vi "Teleop.vi"(10 "Match Info":T1={"Autonomous Elapsed Seconds"=0.0, "TeleOp Elapsed Seconds"=0.0, "Disabled Elapsed Seconds"=0.0, "Visited Autonomous"=FALSE, "Visited TeleOp"=FALSE, "Visited Disabled"=FALSE, "Autonomous Settings"={"Autonomous Style"=enum."Independent", "VI Refnum"=refnum}}, 11 "Call Context":T2) -> ()   [LabVIEW 2013]
doc: "This VI is called for each TeleOp packet received from the DS where the robot is not disabled. It is often used to read from the joysticks and update I/O or to update setpoints for timed control loops. It should complete and return within 20 milliseconds or it may miss DS packets."
uses:
  Robot Global Data.vi
  <vilib>/Rock Robotics/WPI/Joystick/WPI_JoystickDeviceEnum.ctl
  <vilib>/Rock Robotics/WPI/Joystick/WPI_JoystickDevRef.ctl
  <vilib>/Rock Robotics/SystemInterfaces/DIO/FPGA_DIOChannel.ctl
  <vilib>/Rock Robotics/SystemInterfaces/Typedef/FPGA_TypedefDigitalModule.ctl
  <vilib>/Rock Robotics/WPI/DigitalInput/WPI_DigitalInputDevRef.ctl
  <vilib>/Rock Robotics/WPI/RobotDrive/WPI_RobotDriveMecanumDrive_Cartesian.vi
  <vilib>/Rock Robotics/SystemInterfaces/DIO/FPGA_DIORelayChannel.ctl
  <vilib>/Rock Robotics/WPI/Relay/WPI_RelayDirection.ctl
  <vilib>/Rock Robotics/WPI/Relay/WPI_RelayDevRef.ctl
  <vilib>/Rock Robotics/WPI/Relay/WPI_RelayValue.ctl
  <vilib>/Rock Robotics/WPI/DriverStation/WPI_DriverStationMatch Info.ctl
  <vilib>/Rock Robotics/WPI/DriverStation/WPI_DriverStationDerivedRobotMode.ctl
panel:
  out "Right Belt":dbl
  out "Left Belt":dbl
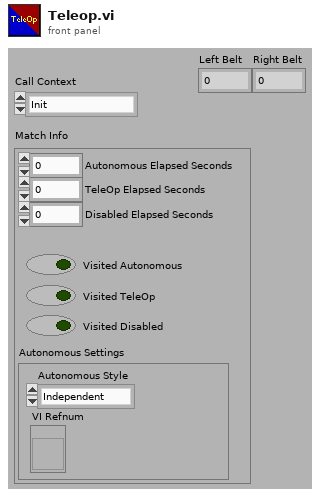
[diagram p1: front panel]
types:
  T1 = typedef "WPI_DriverStationMatch Info.ctl" = cluster{"Autonomous Elapsed Seconds":dbl, "TeleOp Elapsed Seconds":dbl, "Disabled Elapsed Seconds":dbl, "Visited Autonomous":bool, "Visited TeleOp":bool, "Visited Disabled":bool, "Autonomous Settings":cluster{"Autonomous Style":enum16{"Iterative", "Independent"}, "VI Refnum":refnum<vi>}}
  T2 = typedef "WPI_DriverStationDerivedRobotMode.ctl" = enum16{"Init", "Execute", "Stop"}
  T3 = typedef "WPI_RelayDevRef.ctl" = cluster{"DevStatus":errorcluster, "Relay Channel":T4, "Digital Module":T5, "Relay Direction":T6}
  T4 = typedef "FPGA_DIORelayChannel.ctl" = enum8{"Relay 1", "Relay 2", "Relay 3", "Relay 4", "Relay 5", "Relay 6", "Relay 7", "Relay 8", "Invalid"}
  T5 = typedef "FPGA_TypedefDigitalModule.ctl" = enum16{"Digital Module 1", "Digital Module 2"}
  T6 = typedef "WPI_RelayDirection.ctl" = enum16{"Both directions", "Forward only", "Reverse only"}
  T7 = enum16{"Grabbing", "Dropping", "Firing B", "Firing A", "Armed", "Catching"}
  T8 = typedef "WPI_DigitalInputDevRef.ctl" = cluster{"DevStatus":errorcluster, "DIO Channel":T9, "Digital Module":T5}
  T9 = typedef "FPGA_DIOChannel.ctl" = enum8{"DIO 1", "DIO 2", "DIO 3", "DIO 4", "DIO 5", "DIO 6", "DIO 7", "DIO 8", "DIO 9", "DIO 10", "DIO 11", "DIO 12", "DIO 13", "DIO 14", "Invalid"}
  T10 = typedef "WPI_JoystickDevRef.ctl" = cluster{"Device":T11}
  T11 = typedef "WPI_JoystickDeviceEnum.ctl" = enum16{"USB 1", "USB 2", "USB 3", "USB 4", "Kinect 1", "Kinect 2"}
  T12 = typedef "WPI_RobotDriveDevRef.ctl" = cluster{"DevStatus":errorcluster, "Motors[]":T13[], "Square Inputs":bool, "Max Output":dbl, "Isochronous":bool}
  T13 = typedef "WPI_MotorControlDeviceRef.ctl" = cluster{"DeviceStatus":errorcluster, "Type":enum16{"PWM", "CAN"}, "PWM":cluster{"Digital Module":T5, "PWM Channel":T14, "DeadBand":T15}, "CAN":cluster{"Device Number":u8, "Control Mode":T16, "Semaphore":T17, "Max Vout":dbl}, "Invert":bool, "TransformRef":T18, "InvTransformRef":T18}
  T14 = typedef "FPGA_DIOPWMChannel.ctl" = enum8{"PWM 1", "PWM 2", "PWM 3", "PWM 4", "PWM 5", "PWM 6", "PWM 7", "PWM 8", "PWM 9", "PWM 10", "Invalid"}
  T15 = typedef "WPI_PWMDeadband.ctl" = cluster{"Name":string, "maxPositivePwm":i32, "minPositivePwm":i32, "centerPwm":i32, "maxNegativePwm":i32, "minNegativePwm":i32, "angularRange":u16}
  T16 = typedef "WPI_CANJaguar_ControlMode.ctl" = enum8{"Percent VBus", "Current", "Speed", "Position", "Voltage"}
  T17 = typedef "Semaphore RefNum" = refnum<k1>
  T18 = typedef "WPI_PWMTransform_ConPane.ctl" = refnum<vi>
  T19 = typedef "WPI_JoystickButtonState.ctl" = cluster{"Button 1":bool, "Button 2":bool, "Button 3":bool, "Button 4":bool, "Button 5":bool, "Button 6":bool, "Button 7":bool, "Button 8":bool, "Button 9":bool, "Button 10":bool, "Button 11":bool, "Button 12":bool}
  T20 = cluster{"axis 1 (x)":dbl, "axis 2 (y)":dbl, "axis 3 (throttle)":dbl, "axis 4":dbl, "axis 5":dbl, "axis 6":dbl}
  T21 = typedef "WPI_RelayValue.ctl" = enum16{"Off", "On", "Forward", "Reverse"}
  T22 = typedef "WPI_EncoderDevRef.ctl" = cluster{"DevStatus":errorcluster, "EncoderIndex":T23, "CounterIndex":T24, "DistancePerCount":dbl, "Decoding Type":T25}
  T23 = typedef "FPGA_EncoderIdx.ctl" = enum8{"Enc 0", "Enc 1", "Enc 2", "Enc 3", "Invalid"}
  T24 = typedef "FPGA_CounterCtrSystemIndex.ctl" = enum8{"Ctr 0", "Ctr 1", "Ctr 2", "Ctr 3", "Ctr 4", "Ctr 5", "Ctr 6", "Ctr 7", "Invalid"}
  T25 = typedef "WPI_EncoderType.ctl" = enum16{"1x", "2x", "4x"}
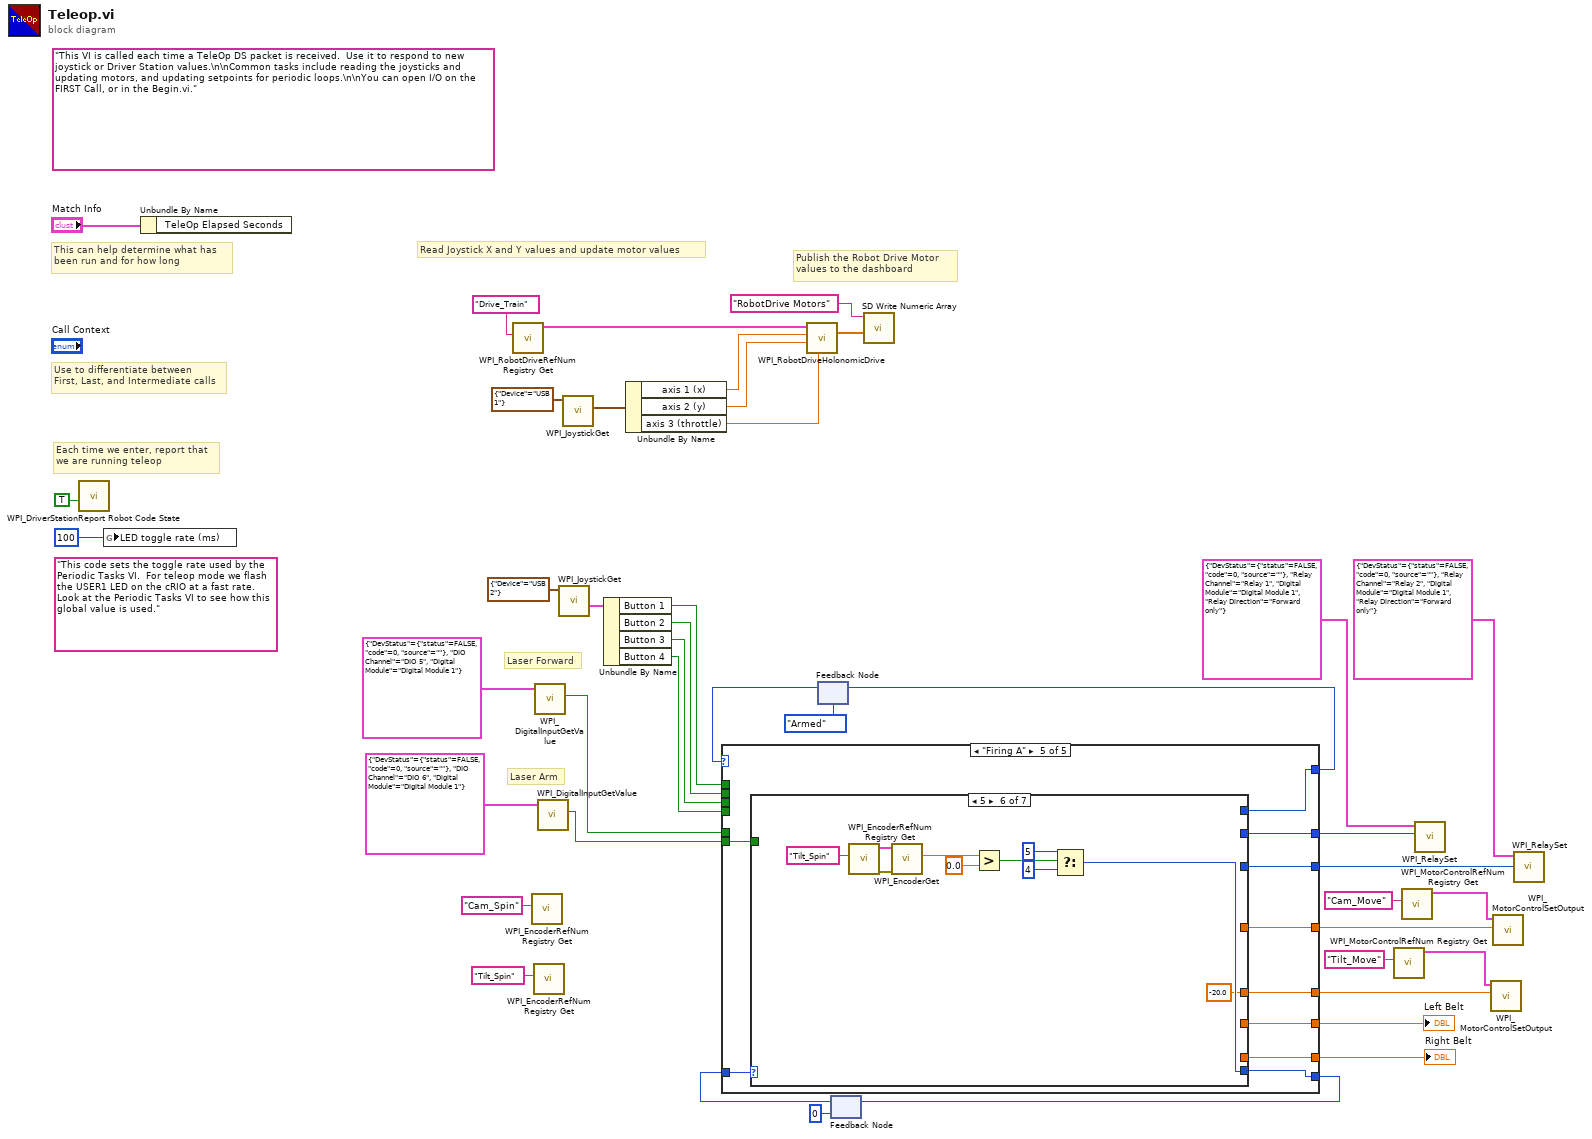
[diagram p0: block diagram]
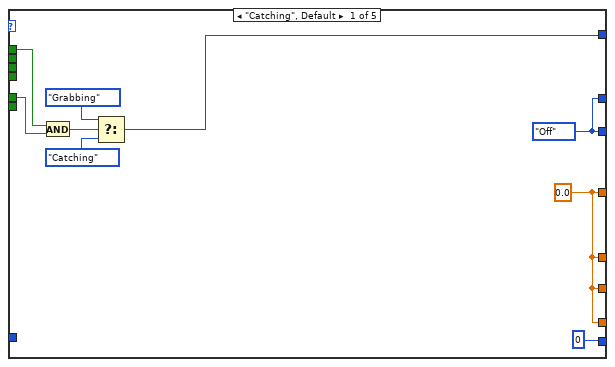
[diagram p2: hidden frame]
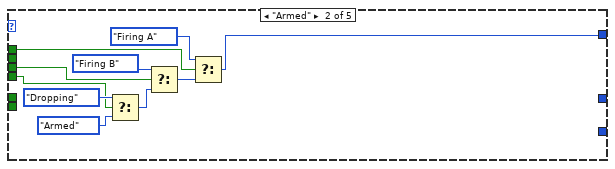
[diagram p3: hidden frame]
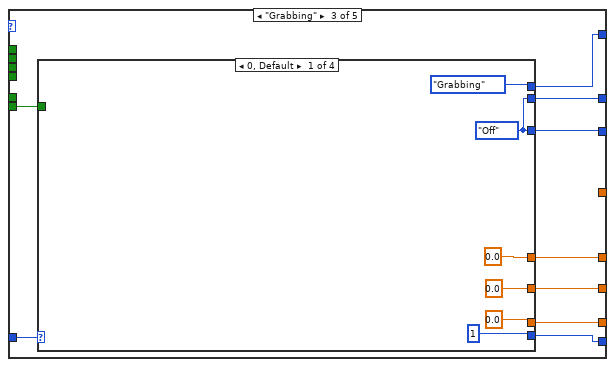
[diagram p4: hidden frame]
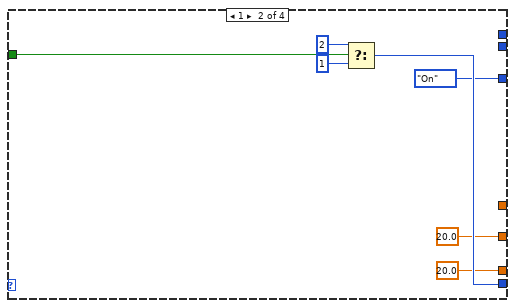
[diagram p5: hidden frame]
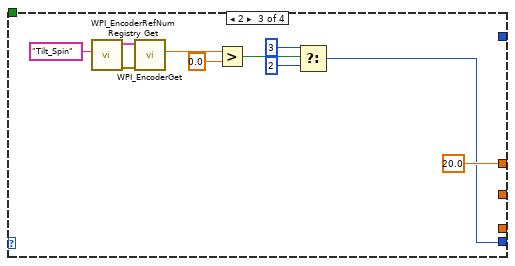
[diagram p6: hidden frame]
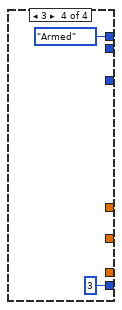
[diagram p7: hidden frame]
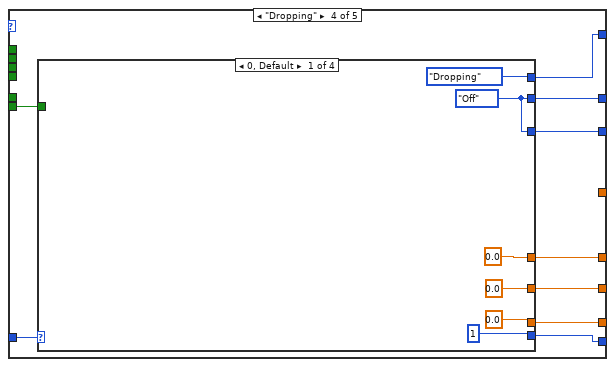
[diagram p8: hidden frame]
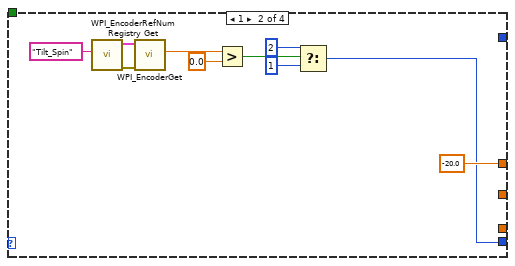
[diagram p9: hidden frame]
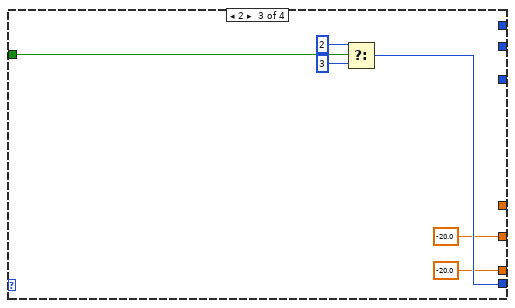
[diagram p10: hidden frame]
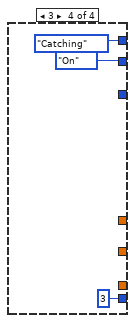
[diagram p11: hidden frame]
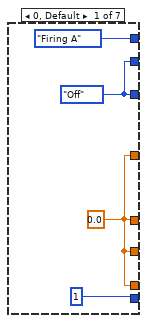
[diagram p12: hidden frame]
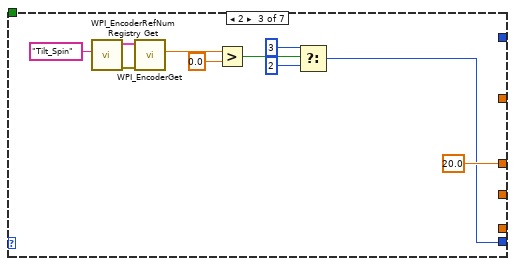
[diagram p14: hidden frame]
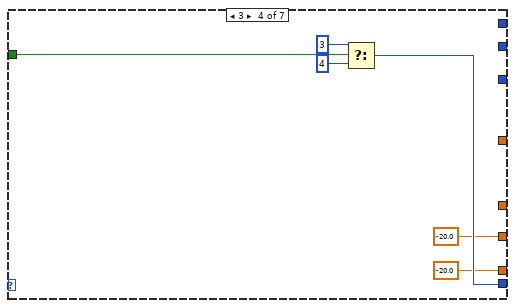
[diagram p15: hidden frame]
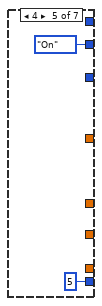
[diagram p16: hidden frame]
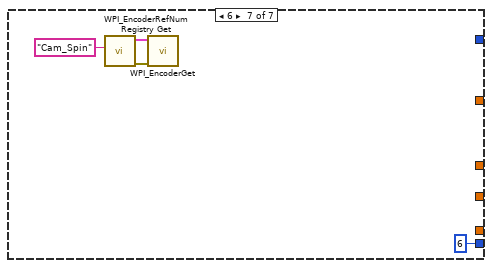
[diagram p17: hidden frame]
diagram:
  (unwired) "This code sets the toggle rate used by the Periodic Tasks VI.  For teleop mode we flash the USER1 LED on the cRIO at a fast rate.  Look at the Periodic Tasks VI to see how this global value is used."
  (unwired) "This VI is called each time a TeleOp DS packet is received.  Use it to respond to new joystick or Driver Station values.\n\nCommon tasks include reading the joysticks and updating motors, and updating setpoints for periodic loops.\n\nYou can open I/O on the FIRST Call, or in the Begin.vi."
  # "Laser Arm"
  # "Laser Forward"
  # "Publish the Robot Drive Motor\nvalues to the dashboard"
  # "Each time we enter, report that\nwe are running teleop"
  # "Use to differentiate between\nFirst, Last, and Intermediate calls"
  # "This can help determine what has\nbeen run and for how long"
  # "Read Joystick X and Y values and update motor values"
  n1 = call <vilib>:"WPI_DriverStationReport Robot Code State.vi"("TeleOp"=TRUE ("Autonomous")) -> ()  [unwired: 10 in, 1 out]
  n2 = global write "Robot Global Data.vi" "LED toggle rate (ms)"(u32 100 ("LED ms toggle rate")) -> ()
  n3 = Unbundle By Name("Match Info") -> ()  [unwired: 1 out]
  n4 = call <vilib>:"WPI_RobotDriveRefNum Registry Get.vi"("refnum name"="Drive_Train") -> ("RobotDriveDevRef"=w40:T12)  [unwired: 1 in, 9 out]
  n5 = call <vilib>:"WPI_EncoderRefNum Registry Get.vi"("refnum name"="Cam_Spin") -> ()  [unwired: 9 in, 2 out]
  n6 = call <vilib>:"WPI_EncoderRefNum Registry Get.vi"("refnum name"="Tilt_Spin") -> ()  [unwired: 9 in, 2 out]
  n7 = call <vilib>:"WPI_DigitalInputGetValue.vi"("DigitalInputDevRef"=T8 {"DevStatus"={"status"=FALSE, "code"=0, "source"=""}, "DIO Channel"=enum."DIO 5", "Digital Module"=enum."Digital Module 1"}) -> ("Value"=w20:bool)  [unwired: 8 in, 2 out]
  n8 = call <vilib>:"WPI_DigitalInputGetValue.vi"("DigitalInputDevRef"=T8 {"DevStatus"={"status"=FALSE, "code"=0, "source"=""}, "DIO Channel"=enum."DIO 6", "Digital Module"=enum."Digital Module 1"}) -> ("Value"=w19:bool)  [unwired: 8 in, 2 out]
  n9 = call <vilib>:"WPI_JoystickGet.vi"("JoystickDevRef"=T10 {"Device"=enum."USB 2"}) -> ("Buttons"=w22:T19)  [unwired: 1 in, 5 out]
  n10 = call <vilib>:"WPI_JoystickGet.vi"("JoystickDevRef"=T10 {"Device"=enum."USB 1"}) -> ("Axes"=w35:T20)  [unwired: 1 in, 5 out]
  n11 = Unbundle By Name(w22) -> ("Button 1"=w21:bool, "Button 2"=w18:bool, "Button 3"=w17:bool, "Button 4"=w16:bool)
  n12 = Unbundle By Name(w35) -> ("axis 1 (x)"=w39:dbl, "axis 2 (y)"=w38:dbl, "axis 3 (throttle)"=w32:dbl)
  n13 = call-poly <vilib>:"WPI_RobotDriveHolonomicDrive.vi"("Rotation"=w32, "Y"=w38, "X"=w39, "RobotDriveDevRef"=w40) -> ("Motor Values"=w33:dbl[])  [unwired: 5 in, 2 out]
  n14 = feedback #1(T7."Armed") -> (w24:T7)
  n15 = feedback #2(0) -> (w15:i32)
  n16 = case shown="\"Firing A\"" w24 {
    tunnel: [w48 w58 w64 w98 w133] -> w23
    tunnel: w21 -> [w51 w52 _ _ _]
    tunnel: w20 -> [w50 _ _ _ _]
    tunnel: w19 -> [_ _ w65 w99 w134]
    tunnel: w18 -> [_ _ _ _ _]
    tunnel: w17 -> [_ w59 _ _ _]
    tunnel: w16 -> [_ w53 _ _ _]
    tunnel: w15 -> [_ _ w70 w104 w139]
    tunnel: [0 _ w67 w101 w136] -> w14
    tunnel: [w44 _ w62 w97 w132] -> w6
    tunnel: [w44 _ w63 w96 w131] -> w5
    tunnel: [w43 _ _ _ w130] -> w4
    tunnel: [w43 _ w66 w100 w135] -> w3
    tunnel: [w43 _ w69 w103 w138] -> w2
    tunnel: [w43 _ w68 w102 w137] -> w1
    frame "Catching", Default {
      w43 = 0.0 ("Output")
      w44 = WPI_RelayValue."Off" ("RelayValue")
      n17 = And(x=w51, y=w50) -> (x .and. y?=w49:bool)
      n18 = Select(t=T7."Grabbing", s=w49, f=T7."Catching") -> (s? t:f=w48:T7)
    }
    frame "Armed" {
      n19 = Select(t=T7."Dropping", s=w53, f=T7."Armed") -> (s? t:f=w61:T7)
      n20 = Select(t=T7."Firing B", s=w59, f=w61) -> (s? t:f=w60:T7)
      n21 = Select(t=T7."Firing A", s=w52, f=w60) -> (s? t:f=w58:T7)
    }
    frame "Grabbing" {
      n22 = case shown="0, Default" w70 {
        tunnel: [0.0 20.0 _ _] -> w69
        tunnel: [0.0 20.0 _ _] -> w68
        tunnel: [1 w80 w84 3] -> w67
        tunnel: [0.0 _ 20.0 _] -> w66
        tunnel: w65 -> [_ w83 _ _]
        tunnel: [T7."Grabbing" _ _ T7."Armed"] -> w64
        tunnel: [w71 WPI_RelayValue."On" ("RelayValue") _ _] -> w63
        tunnel: [w71 _ _ _] -> w62
        frame 0, Default {
          w71 = WPI_RelayValue."Off" ("RelayValue")
        }
        frame 1 {
          n23 = Select(t=2, s=w83, f=1) -> (s? t:f=w80:i32)
        }
        frame 2 {
          n24 = call <vilib>:"WPI_EncoderRefNum Registry Get.vi"("refnum name"="Tilt_Spin") -> ("error out"=w92:errorcluster, "EncoderDevRef"=w91:T22)  [unwired: 9 in]
          n25 = call <vilib>:"WPI_EncoderGet.vi"("error in (no error)"=w92, "EncoderDevRef"=w91) -> ("Distance"=w89:dbl)  [unwired: 4 in, 5 out]
          n26 = Greater?(x=w89, y=0.0) -> (0:w87:bool)
          n27 = Select(t=3, s=w87, f=2) -> (s? t:f=w84:i32)
        }
        frame 3 {
        }
      }
    }
    frame "Dropping" {
      n28 = case shown="0, Default" w104 {
        tunnel: [0.0 _ -20.0 _] -> w103
        tunnel: [0.0 _ -20.0 _] -> w102
        tunnel: [1 w111 w123 3] -> w101
        tunnel: [0.0 -20.0 _ _] -> w100
        tunnel: w99 -> [_ _ w126 _]
        tunnel: [T7."Dropping" _ _ T7."Catching"] -> w98
        tunnel: [w105 _ _ WPI_RelayValue."On" ("RelayValue")] -> w97
        tunnel: [w105 _ _ _] -> w96
        frame 0, Default {
          w105 = WPI_RelayValue."Off" ("RelayValue")
        }
        frame 1 {
          n29 = call <vilib>:"WPI_EncoderRefNum Registry Get.vi"("refnum name"="Tilt_Spin") -> ("error out"=w119:errorcluster, "EncoderDevRef"=w118:T22)  [unwired: 9 in]
          n30 = call <vilib>:"WPI_EncoderGet.vi"("error in (no error)"=w119, "EncoderDevRef"=w118) -> ("Distance"=w116:dbl)  [unwired: 4 in, 5 out]
          n31 = Greater?(x=w116, y=0.0) -> (0:w114:bool)
          n32 = Select(t=2, s=w114, f=1) -> (s? t:f=w111:i32)
        }
        frame 2 {
          n33 = Select(t=2, s=w126, f=3) -> (s? t:f=w123:i32)
        }
        frame 3 {
        }
      }
    }
    frame "Firing A" {
      n34 = case shown="5" w139 {
        tunnel: [w140 _ _ -20.0 _ _ _] -> w138
        tunnel: [w140 _ _ -20.0 _ _ _] -> w137
        tunnel: [1 _ w144 w156 5 w163 6] -> w136
        tunnel: [w140 _ 20.0 _ _ -20.0 _] -> w135
        tunnel: w134 -> [_ _ _ w159 _ _ _]
        tunnel: [T7."Firing A" _ _ _ _ _ _] -> w133
        tunnel: [w141 _ _ _ WPI_RelayValue."On" ("RelayValue") _ _] -> w132
        tunnel: [w141 _ _ _ _ _ _] -> w131
        tunnel: [w140 _ _ _ _ _ _] -> w130
        frame 0, Default {
          w141 = WPI_RelayValue."Off" ("RelayValue")
          w140 = 0.0
        }
        frame 1 {
        }
        frame 2 {
          n35 = call <vilib>:"WPI_EncoderRefNum Registry Get.vi"("refnum name"="Tilt_Spin") -> ("error out"=w152:errorcluster, "EncoderDevRef"=w151:T22)  [unwired: 9 in]
          n36 = call <vilib>:"WPI_EncoderGet.vi"("error in (no error)"=w152, "EncoderDevRef"=w151) -> ("Distance"=w149:dbl)  [unwired: 4 in, 5 out]
          n37 = Greater?(x=w149, y=0.0) -> (0:w147:bool)
          n38 = Select(t=3, s=w147, f=2) -> (s? t:f=w144:i32)
        }
        frame 3 {
          n39 = Select(t=3, s=w159, f=4) -> (s? t:f=w156:i32)
        }
        frame 4 {
        }
        frame 5 {
          n40 = call <vilib>:"WPI_EncoderRefNum Registry Get.vi"("refnum name"="Tilt_Spin") -> ("error out"=w165:errorcluster, "EncoderDevRef"=w166:T22)  [unwired: 9 in]
          n41 = call <vilib>:"WPI_EncoderGet.vi"("error in (no error)"=w165, "EncoderDevRef"=w166) -> ("Distance"=w167:dbl)  [unwired: 4 in, 5 out]
          n42 = Greater?(x=w167, y=0.0) -> (0:w169:bool)
          n43 = Select(t=5, s=w169, f=4) -> (s? t:f=w163:i32)
        }
        frame 6 {
          n44 = call <vilib>:"WPI_EncoderRefNum Registry Get.vi"("refnum name"="Cam_Spin") -> ("error out"=w174:errorcluster, "EncoderDevRef"=w173:T22)  [unwired: 9 in]
          n45 = call <vilib>:"WPI_EncoderGet.vi"("error in (no error)"=w174, "EncoderDevRef"=w173) -> ()  [unwired: 4 in, 6 out]
        }
      }
    }
  }
  "Left Belt" <- w2
  "Right Belt" <- w1
  n46 = feedback-in #1(w23) -> ()
  n47 = feedback-in #2(w14) -> ()
  n48 = call <vilib>:"SD Write Numeric Array.vi"("Numeric Array"=w33, "Name"="RobotDrive Motors") -> ()  [unwired: 8 in, 2 out]
  n49 = call <vilib>:"WPI_MotorControlRefNum Registry Get.vi"("refnum name"="Tilt_Move") -> ("MotorControlDevRef"=w7:T13)  [unwired: 9 in, 1 out]
  n50 = call <vilib>:"WPI_MotorControlRefNum Registry Get.vi"("refnum name"="Cam_Move") -> ("MotorControlDevRef"=w8:T13)  [unwired: 9 in, 1 out]
  n51 = call <vilib>:"WPI_RelaySet.vi"("RelayValue"=w6, "RelayDevRef"=T3 {"DevStatus"={"status"=FALSE, "code"=0, "source"=""}, "Relay Channel"=enum."Relay 1", "Digital Module"=enum."Digital Module 1", "Relay Direction"=enum."Forward only"}) -> ()  [unwired: 8 in, 2 out]
  n52 = call <vilib>:"WPI_MotorControlSetOutput.vi"("Output"=w3, "MotorControlDevRef"=w7) -> ()  [unwired: 7 in, 3 out]
  n53 = call <vilib>:"WPI_MotorControlSetOutput.vi"("Output"=w4, "MotorControlDevRef"=w8) -> ()  [unwired: 7 in, 3 out]
  n54 = call <vilib>:"WPI_RelaySet.vi"("RelayValue"=w5, "RelayDevRef"=T3 {"DevStatus"={"status"=FALSE, "code"=0, "source"=""}, "Relay Channel"=enum."Relay 2", "Digital Module"=enum."Digital Module 1", "Relay Direction"=enum."Forward only"}) -> ()  [unwired: 8 in, 2 out]
